vi "Open FPGA_REF and Init.vi"() -> (0 "error out":errorcluster, 3 "FPGA VI Reference Out":refnum<k20>)   [LabVIEW 2024]
uses:
  <vilib>/FPGAPlugInAG/cRIO-9048/niLvFpga_Open_cRIO-9048.vi
  <vilib>/rvi/interface/common/dynamic/niFpgaDynamicAddResources.vi
  <vilib>/FPGAPlugInAG/Dynamic/niLvFpga_Reset_Dynamic.vi
  <vilib>/Utility/error.llb/Error Cluster From Error Code.vi
  <vilib>/rvi/errors/niLvFpgaAdjustHostInterfaceError.vi
  <vilib>/rvi/interface/common/niFpgaWaitOnOcc.vi
  <vilib>/FPGAPlugInAG/Dynamic/niLvFpga_Run_Dynamic.vi
  <vilib>/rvi/interface/nirviOpenFPGA/nirviOpenFPGA.xnode
  FPGA Bitfiles/depapp_FPGATarget2_FPGAmainsimplifi_Ifa8vhI7MVI.lvbitx
  FPGA Core/FPGA_main_simplified_debug.vi
  <vilib>/rvi/interface/nirviMethod/nirviMethod.xnode
  <vilib>/rvi/interface/nirviReadWriteControl/nirviReadWriteControl.xnode
  <vilib>/rvi/errors/niLvFpgaMergeErrorWithErrorCode.vi
  <vilib>/FPGAPlugInAG/Dynamic/niLvFpga_ConfigureFifo_Dynamic.vi
  <vilib>/FPGAPlugInAG/Dynamic/niLvFpga_StartFifo_Dynamic.vi
  NiFpgaLv.dll
  <vilib>/rvi/interface/Simulation/niFpgaSimulationCallBeginRW.vi
panel:
  out "Triggers FIFO Actual Depth":u32
  out "DMA FIFO Actual Depth":u32
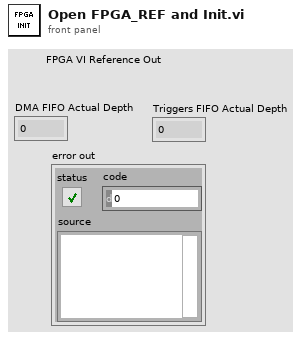
[diagram p1: front panel]
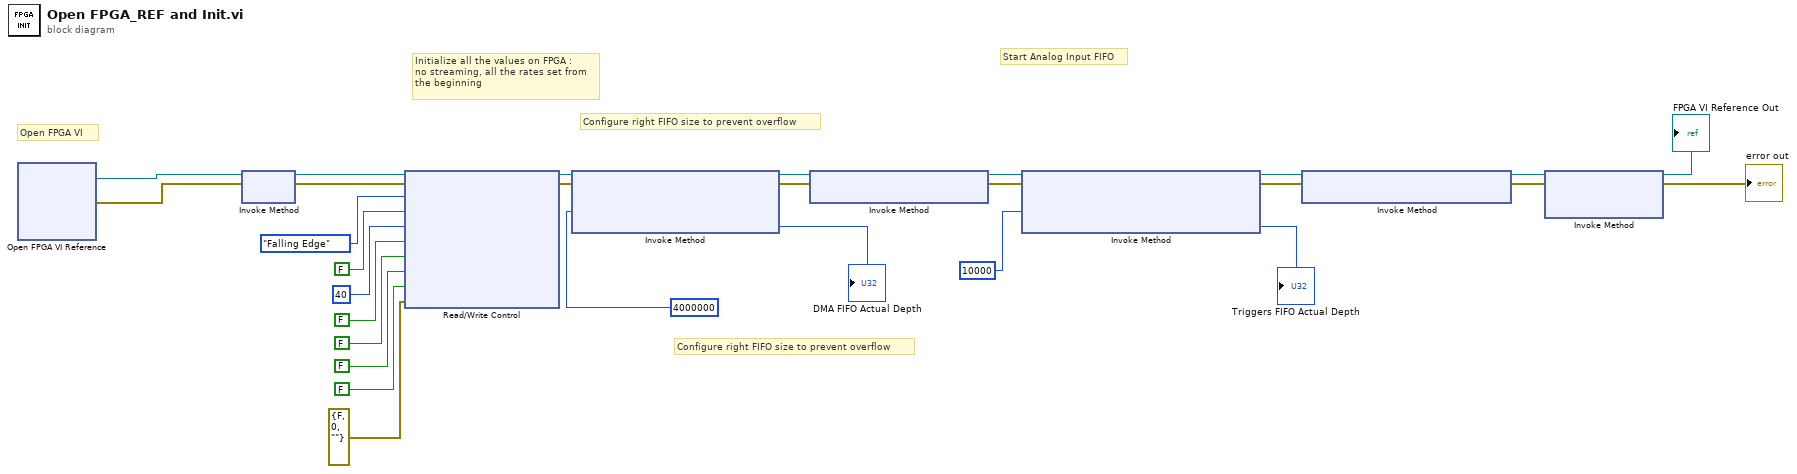
[diagram p0: block diagram]
diagram:
  # "Start Analog Input FIFO"
  # "Configure right FIFO size to prevent overflow"
  # "Configure right FIFO size to prevent overflow"
  # "Initialize all the values on FPGA :\nno streaming, all the rates set from\nthe beginning"
  # "Open FPGA VI"
  n1 = xnode "Open FPGA VI Reference"() -> ("FPGA VI Reference Out"=w11:refnum<k20>, "error out"=w14:errorcluster)  [unwired: 2 in]
  n2 = xnode "Invoke Method"("FPGA VI Reference In"=w11, "error in"=w14) -> ("FPGA VI Reference Out"=w12:refnum<k20>, "error out"=w13:errorcluster)
  n3 = xnode "Read/Write Control"("FPGA VI Reference In"=w12, "error in"=w13, "Type Counter"=enum16{"Falling Edge", "Rising Edge"}."Falling Edge", "First Read"=FALSE, "Actual Loop Period (ticks)"=u32 40, "DMA FIFO Full"=FALSE, "Module Underflow"=FALSE, "Stop"=FALSE, "Finished"=FALSE, "FPGA Error"=errorcluster {"status"=FALSE, "code"=0, "source"=""}) -> ("FPGA VI Reference Out"=w10:refnum<k20>, "error out"=w28:errorcluster)
  n4 = xnode "Invoke Method"("FPGA VI Reference In"=w10, "error in"=w28, "Requested Depth"=u32 4000000) -> ("FPGA VI Reference Out"=w26:refnum<k20>, "error out"=w27:errorcluster, "Actual Depth"=→"DMA FIFO Actual Depth":u32)
  n5 = xnode "Invoke Method"("FPGA VI Reference In"=w26, "error in"=w27) -> ("FPGA VI Reference Out"=w6:refnum<k20>, "error out"=w9:errorcluster)
  n6 = xnode "Invoke Method"("FPGA VI Reference In"=w6, "error in"=w9, "Requested Depth"=u32 10000) -> ("FPGA VI Reference Out"=w5:refnum<k20>, "error out"=w8:errorcluster, "Actual Depth"=→"Triggers FIFO Actual Depth":u32)
  n7 = xnode "Invoke Method"("FPGA VI Reference In"=w5, "error in"=w8) -> ("FPGA VI Reference Out"=w4:refnum<k20>, "error out"=w7:errorcluster)
  n8 = xnode "Invoke Method"("FPGA VI Reference In"=w4, "error in"=w7) -> ("FPGA VI Reference Out"=→"FPGA VI Reference Out":refnum<k20>, "error out"=→"error out":errorcluster)  [unwired: 1 in]
